vi "Raw Data Stream Receiver.vi"(8 "error in (no error)":errorcluster, 11 "Message Queue in":refnum<class "Delacor_lib_QMH_Message Queue.lvclass">) -> ()   [LabVIEW 2015, in "Tool Interface.lvlib"]
uses:
  Tool Interface.lvlib
  <vilib>/Delacor/Delacor QMH/Libraries/Message Queue_class/Delacor_lib_QMH_Message Queue.lvclass
  GLOB - Configuration Options.vi
panel:
  out "error out":errorcluster
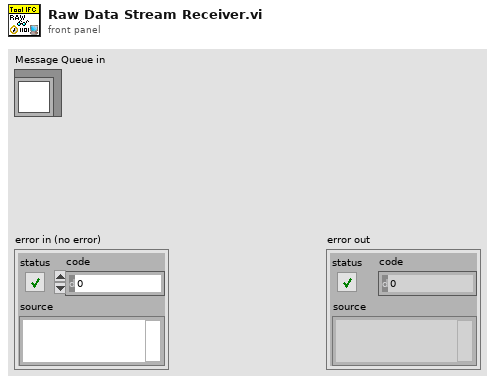
[diagram p1: front panel]
types:
  T1 = typedef "Tool Interface.lvlib/_Loop Ctrl Notifiers Cluster--typedef.ctl" = cluster{"Raw Stream Ctrl":refnum<notifier>}
  T2 = typedef "Tool Interface.lvlib/_HS Data Stream Params Cluster--typedef.ctl" = cluster{"Raw Data Stream Loop cmd":T3, "Data Array DVR ref":refnum<data-value>, "Sample Data notifier":refnum<notifier>, "Block Count Notifier":refnum<notifier>}
  T3 = typedef "Tool Module.lvlib/_HS Data Stream SM enum--typedef.ctl" = enum16{"Idle", "Receive HS Data", "Close Connection"}
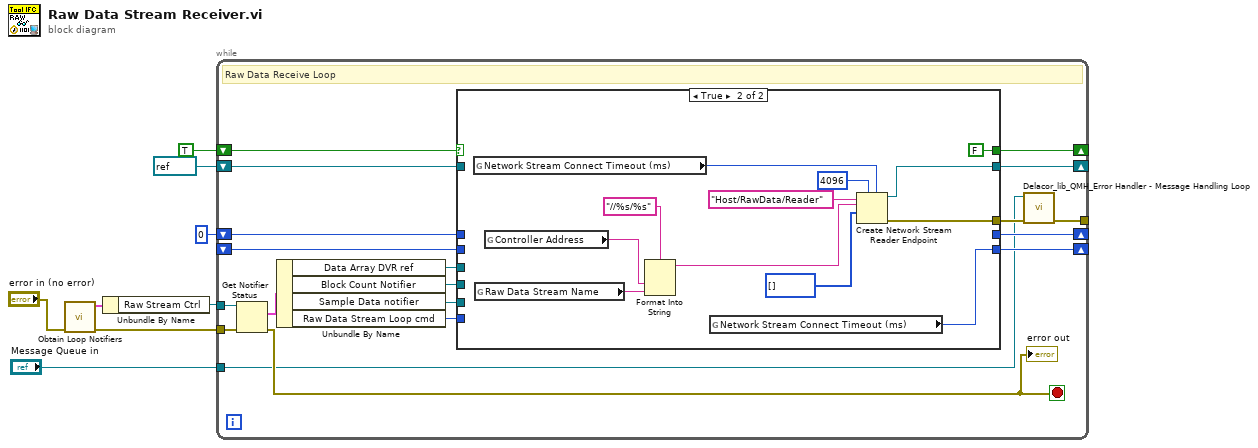
[diagram p0: block diagram]
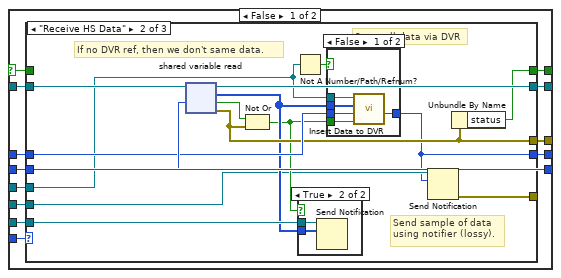
[diagram p2: hidden frame]
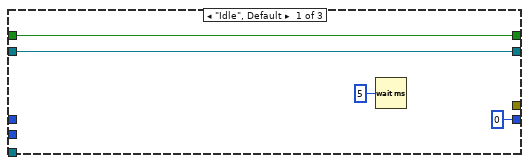
[diagram p3: hidden frame]
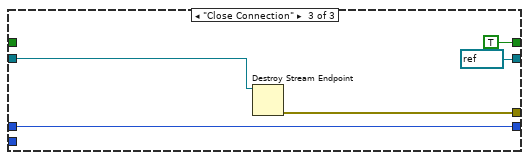
[diagram p6: hidden frame]
diagram:
  n1 = call "Obtain Loop Notifiers.vi"("error in (no error)"="error in (no error)") -> ("error out"=w5:errorcluster, "Loop Ctrl Notifiers Cluster"=w4:T1)  [unwired: 9 in]
  n2 = Unbundle By Name(w4) -> ("Raw Stream Ctrl"=w3:refnum<notifier>)
  n3 = while {
    shift-right: [w26] -> _
    shift-left: TRUE -> [w27]
    shift-right: [w25] -> _
    shift-left: refnum<k21> refnum ("reader name") -> [w24]
    shift-right: [w23] -> _
    shift-left: _ -> [w22]
    tunnel: w3 -> [w21]
    tunnel: w5 -> [w19]
    shift-right: [w17] -> _
    shift-left: u32 0 -> [w18]
    tunnel: "Message Queue in" -> [w11]
    tunnel: [w10] -> _
    stop <- w20 stop-if-true
    # "Raw Data Receive Loop"
    n4 = Get Notifier Status(notifier=w21, error in (no error)=w19) -> (current notification=w16:T2, error out=w20:errorcluster)  [unwired: 3 out]
    "error out" <- w20
    n5 = Unbundle By Name(w16) -> ("Data Array DVR ref"=w13:refnum<data-value>, "Block Count Notifier"=w9:refnum<notifier>, "Sample Data notifier"=w14:refnum<notifier>, "Raw Data Stream Loop cmd"=w15:T3)
    n6 = case shown="True" w27 {
      selector: w27 -> [w37 _]
      tunnel: [w39 FALSE ("status")] -> w26
      tunnel: w15 -> [w38 _]
      tunnel: [w36 w83] -> w12
      tunnel: [w34 w82] -> w25
      tunnel: w24 -> [w35 _]
      tunnel: [w33 w73] -> w23
      tunnel: w22 -> [w33 _]
      tunnel: w18 -> [w32 _]
      tunnel: [w31 _] -> w17
      tunnel: w14 -> [w30 _]
      tunnel: w13 -> [w29 _]
      tunnel: w9 -> [w28 _]
      frame False {
        n7 = case shown="\"Receive HS Data\"" w38 {
          tunnel: [w42 w49 TRUE] -> w39
          tunnel: w37 -> [w42 _ _]
          tunnel: [_ w55 w67] -> w36
          tunnel: w35 -> [w41 w50 w70]
          tunnel: [w41 w51 refnum<k21> refnum ("reader name")] -> w34
          tunnel: w33 -> [_ w57 _]
          tunnel: w32 -> [_ w56 w68]
          tunnel: [u32 0 ("Sample Count out") w47 w68] -> w31
          tunnel: w30 -> [_ w54 _]
          tunnel: w29 -> [_ w45 _]
          tunnel: w28 -> [_ w48 _]
          tunnel: [_ w46 _] -> _
          frame "Idle", Default {
            n8 = Wait (ms)(milliseconds to wait=u32 5) -> ()  [unwired: 1 out]
          }
          frame "Receive HS Data" {
            # "If no DVR ref, then we don't same data."
            # "Store all data via DVR"
            # "Send sample of data\nusing notifier (lossy)."
            n9 = shared-variable-read(w50, w57) -> (w51:refnum<k21>, w55:errorcluster, w58:bool, w53:u32[])  [unwired: 1 in]
            n10 = Not Or(1:w55, 2:w58) -> (0:w52:bool)
            n11 = Not A Number/Path/Refnum?(number/path/refnum=w45) -> (NaN/Path/Refnum?=w44:bool)
            n12 = case shown="True" w52 {
              tunnel: w54 -> [_ w66]
              tunnel: w53 -> [_ w65]
              frame False {
              }
              frame True {
                n13 = Send Notification(notification=w65, notifier=w66) -> ()  [unwired: 1 in, 2 out]
              }
            }
            n14 = case shown="False" w44 {
              tunnel: w56 -> [w63 w64]
              tunnel: w45 -> [w62 _]
              tunnel: w53 -> [w61 _]
              tunnel: w52 -> [w60 _]
              tunnel: [w59 w64] -> w47
              frame False {
                n15 = call "Insert Data to DVR.vi"("Data Available"=w60, "Sample Count"=w63, "New Data"=w61, "Probe Data Array DVR"=w62) -> ("Sample Count out"=w59:u32)  [unwired: 7 in]
              }
              frame True {
              }
            }
            n16 = Send Notification(notification=w47, notifier=w48) -> (error out=w46:errorcluster)  [unwired: 1 in, 1 out]
            n17 = Unbundle By Name(w55) -> ("status"=w49:bool)
          }
          frame "Close Connection" {
            n18 = Destroy Stream Endpoint(11:w70) -> (0:w67:errorcluster)  [unwired: 1 in]
          }
        }
      }
      frame True {
        n19 = global read "GLOB - Configuration Options.vi" "Network Stream Connect Timeout (ms)"() -> (w78:i32)
        n20 = global read "GLOB - Configuration Options.vi" "Raw Data Stream Name"() -> (w72:string)
        n21 = global read "GLOB - Configuration Options.vi" "Controller Address"() -> (w79:string)
        n22 = Format Into String(format string="//%s/%s", w79, w72) -> (resulting string=w75:string)  [unwired: 2 in, 1 out]
        n23 = global read "GLOB - Configuration Options.vi" "Network Stream Connect Timeout (ms)"() -> (w73:i32)
        n24 = Create Network Stream Reader Endpoint(5:w78, 7:4096 ("reader buffer size"), 9:u32[] [], 10:w75, 11:"Host/RawData/Reader" ("reader name")) -> (0:w83:errorcluster, 3:w82:refnum<k21>)  [unwired: 2 in]
      }
    }
    n25 = call-dynamic "Delacor_lib_QMH_Error Handler - Message Handling Loop.vi"("error in (no error)"=w12, "Message Queue in"=w11) -> ("dup error in"=w10:errorcluster)  [unwired: 8 in, 1 out]
  }
